vi "PIDOrPurePursuitSelect.vi"(0 "Distance":dbl, 1 "SensorData":T1, 2 "PurePursuit Gains":T2={"FFV"=0.0055, "FFA"=0.0025, "Vel PID"={"P"=0.005, "I"=0.0, "D"=0.0}}, 3 "Iterations":i16) -> (6 "Graph":cluster{cluster{"x":dbl, "y":dbl}[]}[](graph)=[{[{"x"=0.0, "y"=0.0}, {"x"=6.0, "y"=0.0}, {"x"=12.0, "y"=0.0}, {"x"=18.0, "y"=0.0}, {"x"=24.0, "y"=0.0}, {"x"=30.0, "y"=0.0}, {"x"=36.0, "y"=0.0}, {"x"=42.0, "y"=0.0}, {"x"=48.0, "y"=0.0}, {"x"=54.0, "y"=0.0}, {"x"=55.0, "y"=0.0}, {"x"=60.0, "y"=0.0}]}, {[{"x"=6.595627830179985, "y"=0.002635162832215609}, {"x"=18.59562740071374, "y"=0.005845644049807444}]}, {[{"x"=18.595627540843186, "y"=0.0}]}, {[{"x"=18.595627830179986, "y"=0.002635162832215609}, {"x"=18.333399038985654, "y"=2.4975754526453273}, {"x"=17.558173321891196, "y"=4.883474879741818}, {"x"=16.303831762679355, "y"=7.0560581903418935}, {"x"=14.625195106486284, "y"=8.920373068560945}, {"x"=12.595627830179986, "y"=10.394940008245479}, {"x"=10.303831762679355, "y"=11.415313358374057}, {"x"=7.849969389391829, "y"=11.936897907251494}, {"x"=5.341286270968144, "y"=11.936897907251495}, {"x"=2.8874238976806166, "y"=11.415313358374059}, {"x"=0.5956278301799873, "y"=10.394940008245479}, {"x"=-1.4339394461263106, "y"=8.920373068560949}, {"x"=-3.112576102319383, "y"=7.056058190341894}, {"x"=-4.366917661531224, "y"=4.883474879741821}, {"x"=-5.142143378625682, "y"=2.497575452645332}, {"x"=-5.404372169820015, "y"=0.0026351628322170786}, {"x"=-5.142143378625684, "y"=-2.4923051269808933}, {"x"=-4.366917661531228, "y"=-4.878204554077382}, {"x"=-3.1125761023193865, "y"=-7.050787864677461}, {"x"=-1.4339394461263177, "y"=-8.915102742896513}, {"x"=0.5956278301799793, "y"=-10.389669682581046}, {"x"=2.887423897680614, "y"=-11.410043032709627}, {"x"=5.3412862709681335, "y"=-11.931627581587064}, {"x"=7.849969389391821, "y"=-11.931627581587065}, {"x"=10.303831762679351, "y"=-11.410043032709629}, {"x"=12.595627830179977, "y"=-10.389669682581053}, {"x"=14.625195106486277, "y"=-8.91510274289652}, {"x"=16.30383176267935, "y"=-7.050787864677464}, {"x"=17.558173321891193, "y"=-4.878204554077395}, {"x"=18.33339903898565, "y"=-2.492305126980903}, {"x"=18.595627830179986, "y"=0.00263516283221267}]}, {[{"x"=12326.754773558361, "y"=-12316.860814743844}, {"x"=12057.601746111126, "y"=-9756.040817653475}, {"x"=11261.905942608384, "y"=-7307.140942613652}, {"x"=9974.443087835292, "y"=-5077.189865288984}, {"x"=8251.481486477638, "y"=-3163.647148251028}, {"x"=6168.322828201805, "y"=-1650.1437904310478}, {"x"=3816.0111424787337, "y"=-602.8271511606581}, {"x"=1297.3537376183413, "y"=-67.46999315879293}, {"x"=-1277.571971927846, "y"=-67.46999315879111}, {"x"=-3796.2293767882416, "y"=-602.8271511606563}, {"x"=-6148.541062511309, "y"=-1650.143790431046}, {"x"=-8231.699720787143, "y"=-3163.647148251024}, {"x"=-9954.661322144799, "y"=-5077.189865288982}, {"x"=-11242.12417691789, "y"=-7307.14094261365}, {"x"=-12037.819980420634, "y"=-9756.04081765347}, {"x"=-12306.97300786787, "y"=-12316.860814743843}, {"x"=-12037.819980420634, "y"=-14877.68081183421}, {"x"=-11242.124176917896, "y"=-17326.580686874033}, {"x"=-9954.6613221448, "y"=-19556.531764198706}, {"x"=-8231.69972078715, "y"=-21470.07448123666}, {"x"=-6148.541062511317, "y"=-22983.57783905664}, {"x"=-3796.2293767882443, "y"=-24030.89447832703}, {"x"=-1277.5719719278572, "y"=-24566.251636328896}, {"x"=1297.3537376183326, "y"=-24566.251636328896}, {"x"=3816.011142478731, "y"=-24030.894478327034}, {"x"=6168.322828201795, "y"=-22983.57783905665}, {"x"=8251.481486477633, "y"=-21470.07448123667}, {"x"=9974.44308783529, "y"=-19556.531764198706}, {"x"=11261.90594260838, "y"=-17326.580686874047}, {"x"=12057.601746111126, "y"=-14877.68081183422}, {"x"=12326.754773558361, "y"=-12316.860814743848}]}], 7 "Left Output":dbl, 8 "Right Output":dbl, 9 "Control Mode":T3, 10 "Done?":bool)   [LabVIEW 2020]
uses:
  <vilib>/Rock Robotics/WPI/ThirdParty/REV Robotics/REVLib/Typedef/Spark MAX Control Type.ctl
  Configuration/Constants.vi
panel:
  in  "PurePursuit?":bool=TRUE
  in  "Threshold":dbl=0.5 format="%#_13g"
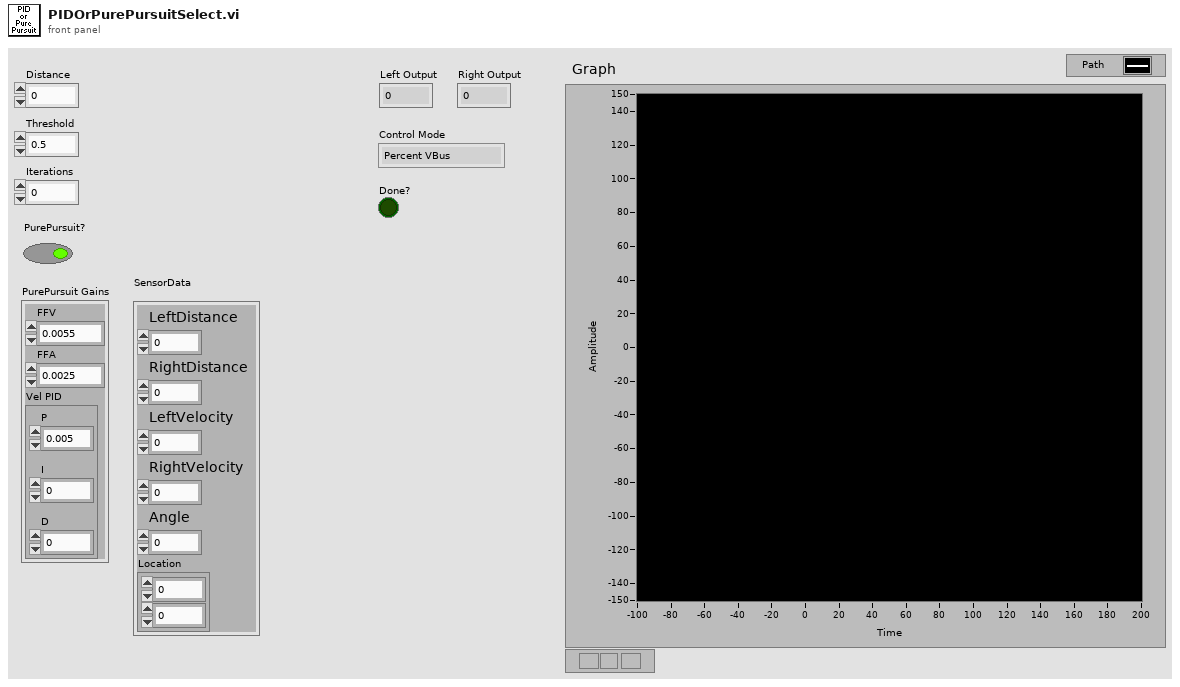
[diagram p1: front panel]
types:
  T1 = cluster{"LeftDistance":dbl, "RightDistance":dbl, "LeftVelocity":dbl, "RightVelocity":dbl, "Angle":dbl, "Location":cluster{dbl, dbl}}
  T2 = cluster{"FFV":dbl, "FFA":dbl, "Vel PID":cluster{"P":dbl, "I":dbl, "D":dbl}}
  T3 = typedef "Spark MAX Control Type.ctl" = enum16{"Percent VBus", "Voltage", "Velocity", "Position", "Smart Motion", "Current", "Smart Velocity"}
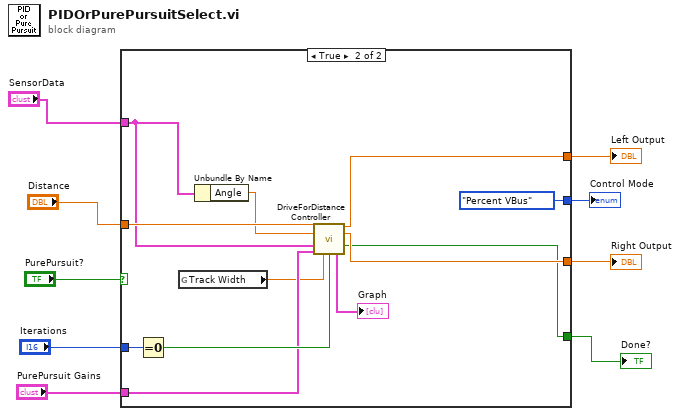
[diagram p0: block diagram]
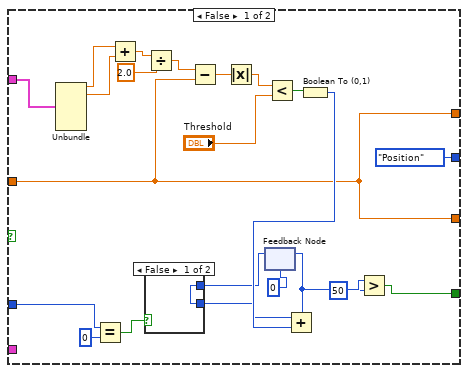
[diagram p2: hidden frame]
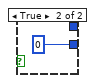
[diagram p3: hidden frame]
diagram:
  n1 = case shown="True" "PurePursuit?" {
    tunnel: [w20 w38] -> w9
    tunnel: "Iterations" -> [w15 w44]
    tunnel: "Distance" -> [w10 w45]
    tunnel: [Spark_MAX_Control_Type."Position" ("Control Mode") Spark_MAX_Control_Type."Percent VBus" ("Control Mode")] -> w6
    tunnel: "SensorData" -> [w11 w35]
    tunnel: [w10 w41] -> w4
    tunnel: [w10 w40] -> w3
    tunnel: "PurePursuit Gains" -> [_ w37]
    frame False {
      n2 = Unbundle(w11) -> ("LeftDistance"=w14:dbl, "RightDistance"=w13:dbl)  [unwired: 4 out]
      n3 = Equal?(x=w15, y=0) -> (x = y?=w18:bool)
      n4 = Add(x=w14, y=w13) -> (x+y=w31:dbl)
      n5 = Divide(x=w31, y=2.0) -> (x/y=w29:dbl)
      n6 = Subtract(x=w29, y=w10) -> (x-y=w28:dbl)
      n7 = Absolute Value(x=w28) -> (abs(x)=w27:dbl)
      n8 = feedback #1(0) -> (w16:i32)
      n9 = case shown="False" w18 {
        tunnel: [w32 0] -> w17
        tunnel: w16 -> [w32 _]
        frame False {
        }
        frame True {
        }
      }
      n10 = Less?(x=w27, y="Threshold") -> (x < y?=w25:bool)
      n11 = Boolean To (0,1)(Boolean=w25) -> (0, 1=w23:i16)
      n12 = Add(x=w17, y=w23) -> (x+y=w22:i32)
      n13 = feedback-in #1(w22) -> ()
      n14 = Greater?(x=w22, y=50) -> (0:w20:bool)
    }
    frame True {
      n15 = Equal To 0?(x=w44) -> (x = 0?=w43:bool)
      n16 = global read "Constants.vi" "Track Width"() -> (w36:dbl)
      n17 = Unbundle By Name(w35) -> ("Angle"=w34:dbl)
      n18 = call "DriveForDistanceController.vi"("Distance"=w45, "Angle"=w34, "SensorData"=w35, "Gains"=w37, "Trackwidth"=w36, "Reset"=w43) -> ("Left Speed"=w41:dbl, "Right Speed"=w40:dbl, "Done"=w38:bool, "Graph"=→"Graph":cluster{cluster{"x":dbl, "y":dbl}[]}[])  [unwired: 5 in, 1 out]
    }
  }
  "Left Output" <- w4
  "Right Output" <- w3
  "Control Mode" <- w6
  "Done?" <- w9
